vi "Shift and prune points.vi"   [LabVIEW 2014]
uses:
  Labby Bird/Labby Bird/Labby bird-Support.llb/Global-1.vi
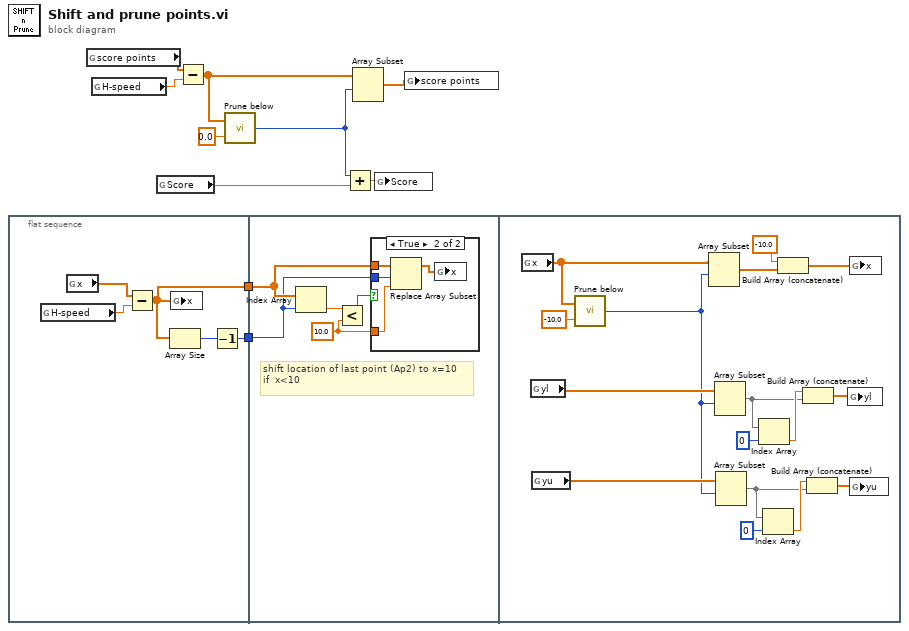
[diagram p0: block diagram]
diagram:
  n1 = flat-sequence {
    tunnel: [w11] -> w10
    tunnel: [w15] -> w9
    tunnel: w10 -> [w19]
    tunnel: w9 -> [w20]
    frame #0 {
      n2 = global read "Global-1.vi" "H-speed"() -> (w13:dbl)
      n3 = global read "Global-1.vi" "x"() -> (w14:dbl[])
      n4 = Subtract(x=w14, y=w13) -> (x-y=w15:dbl[])
      n5 = Array Size(array=w15) -> (size(s)=w12:i32)
      n6 = global write "Global-1.vi" "x"(w15) -> ()
      n7 = Decrement(x=w12) -> (x-1=w11:i32)
    }
    frame #1 {
      w16 = 10.0 ("y")
      # "shift location of last point (Ap2) to x=10\nif  x<10"
      n8 = Index Array(array=w20, index=w19) -> (element=w18:dbl)
      n9 = Less?(x=w18, y=w16) -> (x < y?=w17:bool)
      n10 = case shown="True" w17 {
        tunnel: w20 -> [_ w24]
        tunnel: w19 -> [_ w22]
        tunnel: w16 -> [_ w21]
        frame False {
        }
        frame True {
          n11 = Replace Array Subset(array=w24, new element=w21, index=w22) -> (w23:dbl[])
          n12 = global write "Global-1.vi" "x"(w23) -> ()
        }
      }
    }
    frame #2 {
      n13 = global read "Global-1.vi" "x"() -> (w27:dbl[])
      n14 = global read "Global-1.vi" "yl"() -> (w39:dbl[])
      n15 = global read "Global-1.vi" "yu"() -> (w38:dbl[])
      n16 = call "Prune below.vi"("lower limit"=-10.0, "Array in"=w27) -> ("Index out"=w26:i32)
      n17 = Array Subset(array=w27, index=w26) -> (w37:dbl[])  [unwired: 1 in]
      n18 = Array Subset(array=w39, index=w26) -> (w34:dbl[])  [unwired: 1 in]
      n19 = Array Subset(array=w38, index=w26) -> (w29:dbl[])  [unwired: 1 in]
      n20 = Index Array(array=w34, index=0) -> (element=w35:dbl)
      n21 = Index Array(array=w29, index=0) -> (element=w31:dbl)
      n22 = Build Array (concatenate)(-10.0, w37) -> (w28:dbl[])
      n23 = Build Array (concatenate)(w35, w34) -> (w33:dbl[])
      n24 = Build Array (concatenate)(w31, w29) -> (w30:dbl[])
      n25 = global write "Global-1.vi" "yl"(w33) -> ()
      n26 = global write "Global-1.vi" "x"(w28) -> ()
      n27 = global write "Global-1.vi" "yu"(w30) -> ()
    }
  }
  n28 = global read "Global-1.vi" "score points"() -> (w4:dbl[])
  n29 = global read "Global-1.vi" "H-speed"() -> (w5:dbl)
  n30 = global read "Global-1.vi" "Score"() -> (w6:dbl)
  n31 = Subtract(x=w4, y=w5) -> (x-y=w3:dbl[])
  n32 = call "Prune below.vi"("lower limit"=0.0, "Array in"=w3) -> ("Index out"=w2:i32)
  n33 = Add(x=w2, y=w6) -> (x+y=w7:dbl)
  n34 = Array Subset(array=w3, index=w2) -> (w8:dbl[])  [unwired: 1 in]
  n35 = global write "Global-1.vi" "Score"(w7) -> ()
  n36 = global write "Global-1.vi" "score points"(w8) -> ()
